vi "Analysis_worker.vi"(5 "Leftover data in":T1, 6 "error in":errorcluster, 7 "Analysis parameters":T3, 8 "Data in":T1, 9 "Analysis in":T4) -> (0 "error out":errorcluster, 2 "Data out":T1, 3 "Analysis out":T4, 4 "Leftover data out":T1)   [LabVIEW 2010]
uses:
  typedefs/analysis_channels_array.ctl
  typedefs/analysis_cluster.ctl
  typedefs/experiment_mode_enum.ctl
  typedefs/data_cluster.ctl
  <vilib>/Analysis/NI_AALBase.lvlib
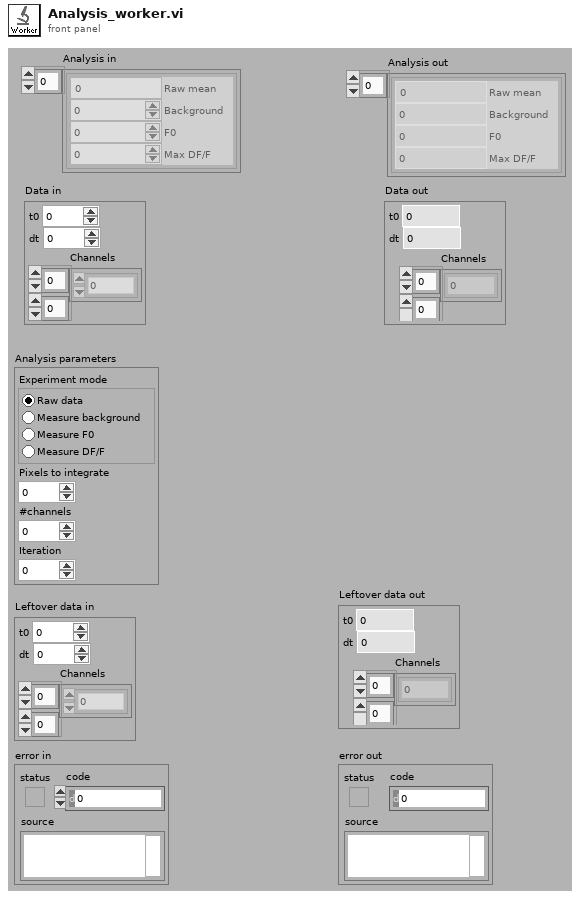
[diagram p1: front panel]
types:
  T1 = typedef "data_cluster.ctl" = cluster{"t0":dbl, "dt":dbl, "Channels":dbl[][]}
  T2 = typedef "experiment_mode_enum.ctl" = enum32{"Raw data", "Measure background", "Measure F0", "Measure DF/F"}
  T3 = cluster{"Experiment mode":T2, "Pixels to integrate":i32, "#channels":i32, "Iteration":i32}
  T4 = typedef "analysis_channels_array.ctl" = T5[]
  T5 = typedef "analysis_cluster.ctl" = cluster{"Raw mean":dbl, "Background":dbl, "F0":dbl, "Max DF/F":dbl}
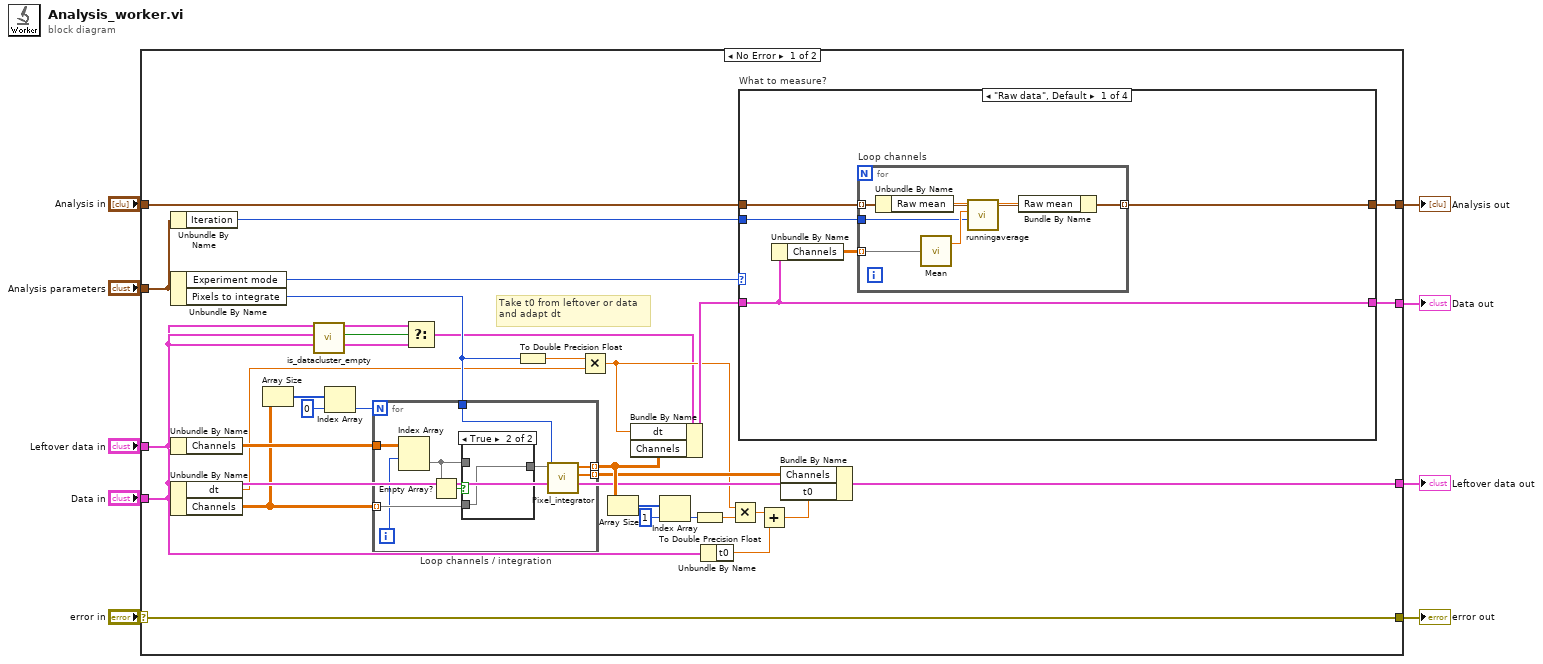
[diagram p0: block diagram]
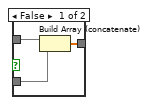
[diagram p2: hidden frame]
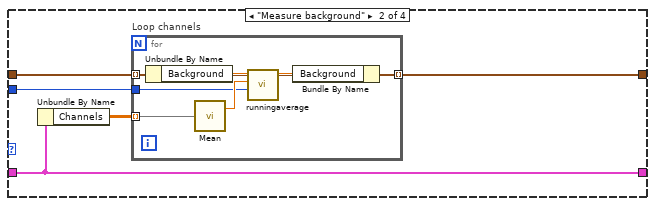
[diagram p3: hidden frame]
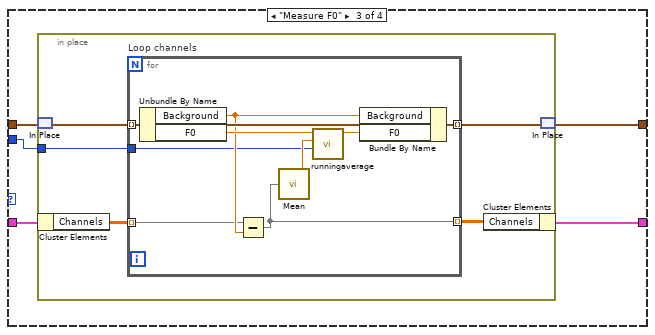
[diagram p4: hidden frame]
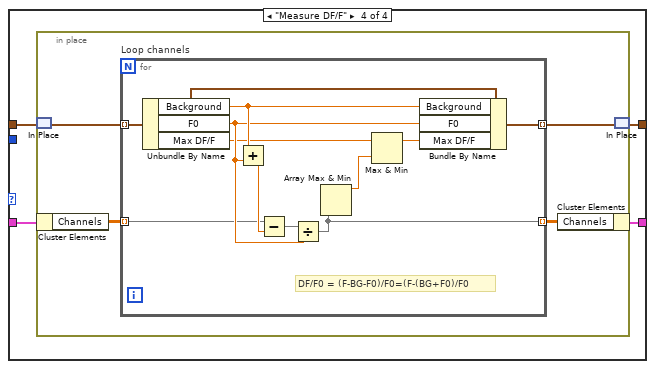
[diagram p5: hidden frame]
diagram:
  n1 = case shown="No Error" "error in" {
    selector: "error in" -> [w22 w118]
    tunnel: "Data in" -> [w19 w117]
    tunnel: [w37 w117] -> w2
    tunnel: "Analysis in" -> [w40 w119]
    tunnel: "Analysis parameters" -> [w36 _]
    tunnel: "Leftover data in" -> [w20 w116]
    tunnel: [w38 w119] -> w7
    tunnel: [w23 w116] -> w3
    tunnel: [w22 w118] -> w1
    frame No Error {
      # "Take t0 from leftover or data\nand adapt dt"
      n2 = Unbundle By Name(w36) -> ("Iteration"=w35:i32)
      n3 = Unbundle By Name(w36) -> ("Experiment mode"=w39:T2, "Pixels to integrate"=w33:i32)
      n4 = Unbundle By Name(w20) -> ("Channels"=w34:dbl[][])
      n5 = Unbundle By Name(w19) -> ("dt"=w16:dbl, "Channels"=w13:dbl[][])
      n6 = Array Size(array=w13) -> (size(s)=w12:i32[])
      n7 = call "is_datacluster_empty.vi"("Data_cluster"=w20) -> ("Is empty?"=w21:bool)  [unwired: 10 in]
      n8 = Index Array(array=w12, index=0) -> (element=w10:i32)
      n9 = for "Loop channels / integration" {
        N: w10 -> [_]
        tunnel: w33 -> [w49]
        tunnel: [w45] -> w31 mode=indexing
        tunnel: [w48] -> w28 mode=indexing
        tunnel: w13 -> [w47] mode=indexing
        tunnel: w34 -> [w43]
        i -> [w41]
        n10 = Index Array(array=w43, index (row)=w41) -> (element=w42:dbl[])  [unwired: 1 in]
        n11 = Empty Array?(array=w42) -> (empty?=w44:bool)
        n12 = case shown="True" w44 {
          tunnel: w42 -> [w52 _]
          tunnel: w47 -> [w51 w53]
          tunnel: [w50 w53] -> w46
          frame False {
            n13 = Build Array (concatenate)(w52, w51) -> (w50:dbl[])
          }
          frame True {
          }
        }
        n14 = call "Pixel_integrator.vi"("Pixels to integrate"=w49, "Data in"=w46) -> ("Leftover data out"=w48:dbl[], "Data out"=w45:dbl[])  [unwired: 6 in]
      }
      n15 = Select(t=w19, s=w21, f=w20) -> (s? t:f=w15:T1)
      n16 = To Double Precision Float(number=w33) -> (double precision float=w14:dbl)
      n17 = Multiply(x=w14, y=w16) -> (x*y=w17:dbl)
      n18 = Array Size(array=w31) -> (size(s)=w30:i32[])
      n19 = Bundle By Name(cluster=w15, "dt"=w17, "Channels"=w31) -> (w32:T1)
      n20 = Index Array(array=w30, index=1) -> (element=w25:i32)
      n21 = To Double Precision Float(number=w25) -> (double precision float=w18:dbl)
      n22 = Unbundle By Name(w19) -> ("t0"=w26:dbl)
      n23 = Multiply(x=w17, y=w18) -> (x*y=w27:dbl)
      n24 = case "What to measure?" shown="\"Raw data\", Default" w39 {
        tunnel: [w55 w68 w81 w99] -> w37
        tunnel: w40 -> [w58 w70 w80 w98]
        tunnel: [w57 w69 w79 w97] -> w38
        tunnel: w32 -> [w55 w68 w82 w100]
        tunnel: w35 -> [w56 w66 w78 _]
        frame "Raw data", Default {
          n25 = Unbundle By Name(w55) -> ("Channels"=w54:dbl[][])
          n26 = for "Loop channels" {
            tunnel: w58 -> [w62] mode=indexing
            tunnel: [w61] -> w57 mode=indexing
            tunnel: w56 -> [w60]
            tunnel: w54 -> [w59] mode=indexing
            n27 = Unbundle By Name(w62) -> ("Raw mean"=w65:dbl)
            n28 = call <vilib>:"Mean.vi"("X"=w59) -> ("mean"=w64:dbl)  [unwired: 1 out]
            n29 = call "runningaverage.vi"("Iteration"=w60, "New value"=w64, "Average in"=w65) -> ("Average out"=w63:dbl)  [unwired: 8 in]
            n30 = Bundle By Name(cluster=w62, "Raw mean"=w63) -> (w61:T5)
          }
        }
        frame "Measure background" {
          n31 = Unbundle By Name(w68) -> ("Channels"=w67:dbl[][])
          n32 = for "Loop channels" {
            tunnel: w70 -> [w74] mode=indexing
            tunnel: [w73] -> w69 mode=indexing
            tunnel: w67 -> [w72] mode=indexing
            tunnel: w66 -> [w71]
            n33 = Unbundle By Name(w74) -> ("Background"=w77:dbl)
            n34 = call <vilib>:"Mean.vi"("X"=w72) -> ("mean"=w76:dbl)  [unwired: 1 out]
            n35 = call "runningaverage.vi"("Iteration"=w71, "New value"=w76, "Average in"=w77) -> ("Average out"=w75:dbl)  [unwired: 8 in]
            n36 = Bundle By Name(cluster=w74, "Background"=w75) -> (w73:T5)
          }
        }
        frame "Measure F0" {
          n37 = in-place {
            in-place-border: w78 -> [w83]
            n38 = in-place-match #1(w80) -> (w85:T4)
            n39 = in-place-cluster #2(w82) -> ("Channels"=w87:dbl[][])
            n40 = for "Loop channels" {
              tunnel: w85 -> [w96] mode=indexing
              tunnel: [w95] -> w84 mode=indexing
              tunnel: w87 -> [w90] mode=indexing
              tunnel: [w89] -> w86 mode=indexing
              tunnel: w83 -> [w88]
              n41 = Unbundle By Name(w96) -> ("Background"=w91:dbl, "F0"=w93:dbl)
              n42 = Subtract(x=w90, y=w91) -> (x-y=w89:dbl[])
              n43 = call <vilib>:"Mean.vi"("X"=w89) -> ("mean"=w92:dbl)  [unwired: 1 out]
              n44 = call "runningaverage.vi"("Iteration"=w88, "New value"=w92, "Average in"=w93) -> ("Average out"=w94:dbl)  [unwired: 8 in]
              n45 = Bundle By Name(cluster=w96, "Background"=w91, "F0"=w94) -> (w95:T5)
            }
            n46 = in-place-cluster #2("Channels"=w86) -> (w81:T1)
            n47 = in-place-match #1(w84) -> (w79:T4)
          }
        }
        frame "Measure DF/F" {
          n48 = in-place {
            n49 = in-place-match #3(w98) -> (w102:T4)
            n50 = in-place-cluster #4(w100) -> ("Channels"=w104:dbl[][])
            n51 = for "Loop channels" {
              tunnel: w102 -> [w115] mode=indexing
              tunnel: [w114] -> w101 mode=indexing
              tunnel: w104 -> [w106] mode=indexing
              tunnel: [w105] -> w103 mode=indexing
              # "DF/F0 = (F-BG-F0)/F0=(F-(BG+F0)/F0"
              n52 = Unbundle By Name(w115) -> ("Background"=w112:dbl, "F0"=w111:dbl, "Max DF/F"=w110:dbl)
              n53 = Add(x=w112, y=w111) -> (x+y=w113:dbl)
              n54 = Subtract(x=w106, y=w113) -> (x-y=w107:dbl[])
              n55 = Divide(x=w107, y=w111) -> (x/y=w105:dbl[])
              n56 = Array Max & Min(array=w105) -> (max value=w109:dbl)  [unwired: 3 out]
              n57 = Max & Min(x=w110, y=w109) -> (max(x,y)=w108:dbl)  [unwired: 1 out]
              n58 = Bundle By Name(cluster=w115, "Background"=w112, "F0"=w111, "Max DF/F"=w108) -> (w114:T5)
            }
            n59 = in-place-cluster #4("Channels"=w103) -> (w99:T1)
            n60 = in-place-match #3(w101) -> (w97:T4)
          }
        }
      }
      n61 = Add(x=w27, y=w26) -> (x+y=w24:dbl)
      n62 = Bundle By Name(cluster=w19, "Channels"=w28, "t0"=w24) -> (w23:T1)
    }
    frame Error {
    }
  }
  "error out" <- w1
  "Analysis out" <- w7
  "Data out" <- w2
  "Leftover data out" <- w3
